vi "CRYAppend data or results file.vi"(3 "Excel path":path, 4 "Is results? (F)":bool, 5 "New/Append":string, 6 "Comment":string, 7 "Format info":T1, 8 "data format":u16, 9 "Datafile path":path, 10 "Curves list to save":string[](array[string]), 11 "Data/Wave(if true=wave)?":bool) -> (1 "error out":errorcluster)   [LabVIEW 2013]
uses:
  Data/CRYData & result stacks global.vi
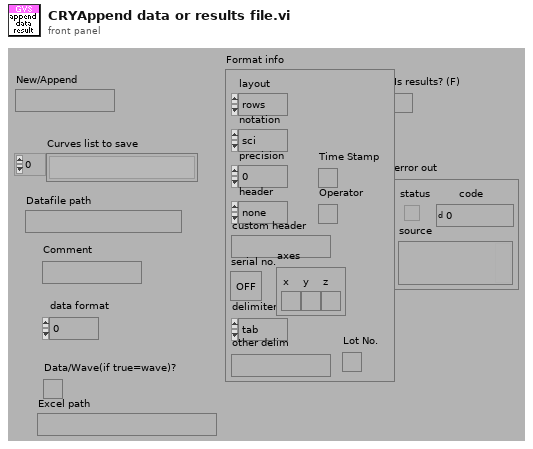
[diagram p1: front panel]
types:
  T1 = cluster{"layout":enum16{"rows", "columns"}, "notation":enum16{"sci", "float"}, "precision":i32, "header":enum16{"none", "standard", "custom"}, "custom header":string, "serial no.":bool, "delimiter":enum16{"tab", "comma", "space", "other"}, "other delim":string, "axes":cluster{"x":bool, "y":bool, "z":bool}, "Lot No.":bool, "Operator":bool, "Time Stamp":bool}
  T2 = enum16{"open", "open or create", "create or replace", "create"}
  T3 = cluster{"Datafile path":path, "file size (bytes)":i32}
  T4 = cluster{"Datafile path":path, "file size (bytes)":i32}[]
  T5 = enum16{"OK", "Yes", "YesNo", "YesNoCancel", "ReplaceAppend"}
  T6 = typedef "CRYData Cluster.ctl" = cluster{"Name":string, "Curve":cluster{"x":dbl, "y":dbl, "z":dbl}[], "X data":u16, "Y data":u16, "Z data":u16, "X axis":u16, "Y axis":u16, "Z axis":u16, "X unit":string, "Y unit":string, "Z unit":string, "X dB ref":dbl, "Y dB ref":dbl, "Z dB ref":dbl, "single val":bool, "protected":bool, "display X":bool, "display Y":bool, "display Z":bool, "Test Info":string, "Step No.":i32, "Plot Settings":cluster{"Color":u32, "Interpolation":u8, "Point Style":u8, "Line Style":u8, "Point Color":u32, "Line Width":u8, "Bar Plot Style":u8, "Fill To":i16}, "AutoProtect":bool}
  T7 = typedef "CRYResult Cluster.ctl" = cluster{"Name":string, "Margin":dbl, "unit":string, "Verdict":bool, "Limit":string, "Max/Min":string, "protected":bool, "Step No.":i32, "Test Info":string, "AutoProtect":bool}
  T8 = typedef "CRYWaveform Cluster.ctl" = cluster{"Waveform":cluster{"X0":dbl, "dX":dbl, "Y":sgl[]}, "X data":u16, "Y data":u16, "Y axis":u16, "X unit":string, "Y unit":string, "Y dB ref":dbl, "display Y":bool, "display X":bool, "Overload?":bool, "Test Info":string, "Step No.":i32, "Name":string, "protected":bool, "Sqc history":string[], "Signal Channel ID":i32, "Plot Settings":cluster{"Color":u32, "Interpolation":u8, "Point Style":u8, "Line Style":u8, "Point Color":u32, "Line Width":u8, "Bar Plot Style":u8, "Fill To":i16}, "AutoProtect":bool}
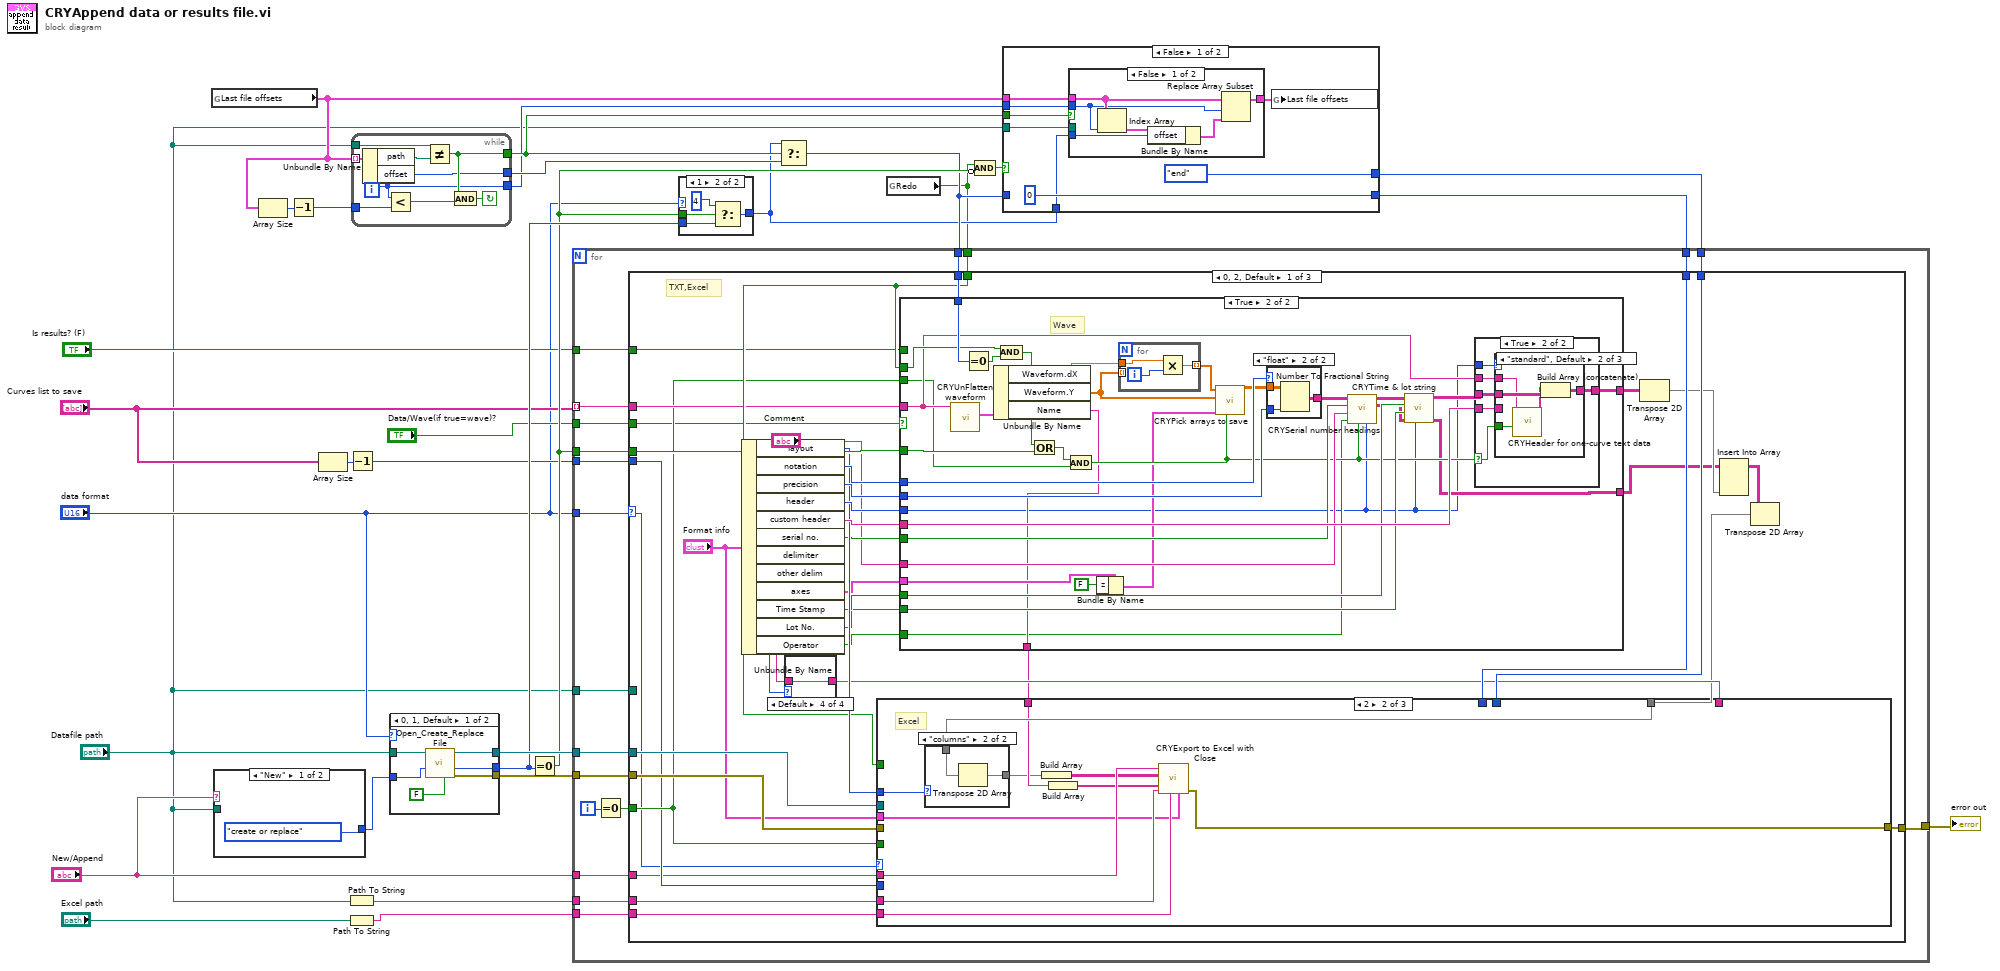
[diagram p0: block diagram]
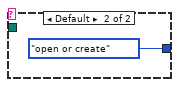
[diagram p2: hidden frame]
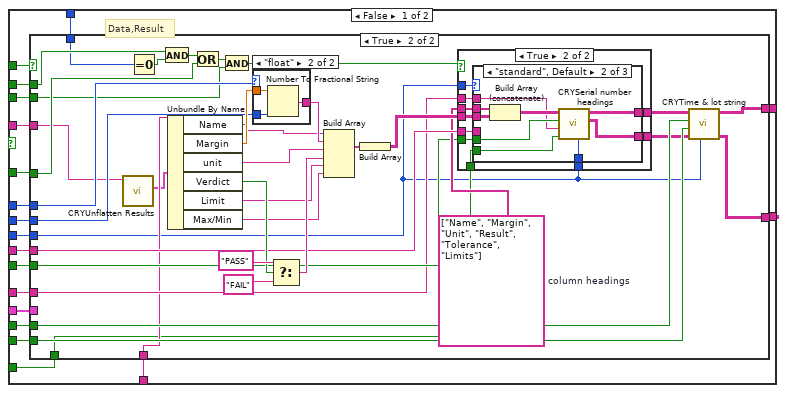
[diagram p4: hidden frame]
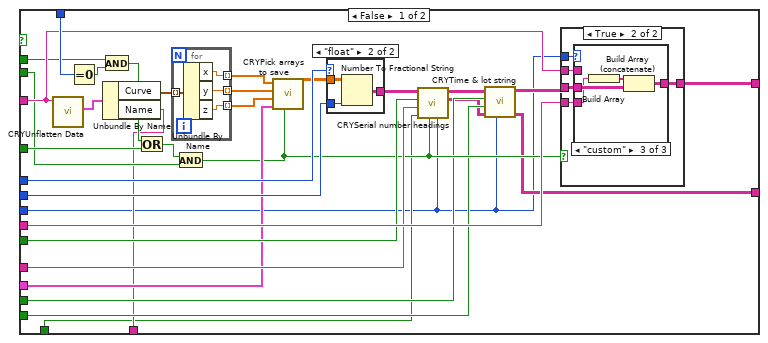
[diagram p5: hidden frame]
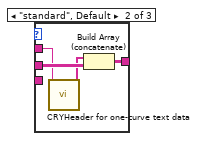
[diagram p8: hidden frame]
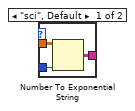
[diagram p9: hidden frame]
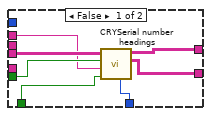
[diagram p10: hidden frame]
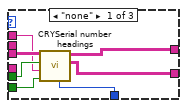
[diagram p11: hidden frame]
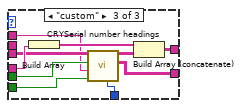
[diagram p12: hidden frame]
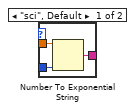
[diagram p13: hidden frame]
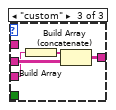
[diagram p16: hidden frame]
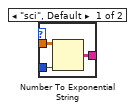
[diagram p17: hidden frame]
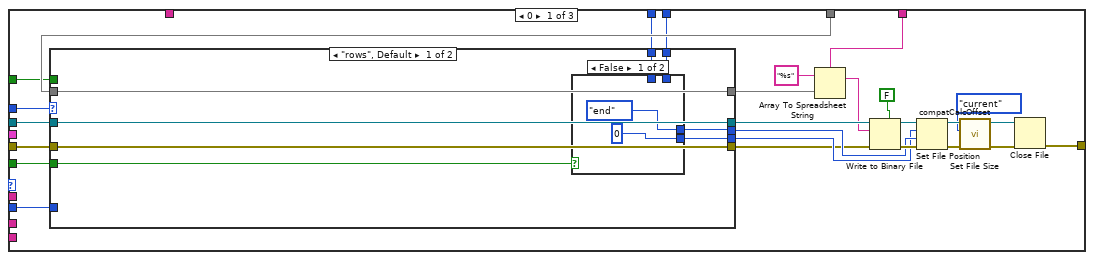
[diagram p18: hidden frame]
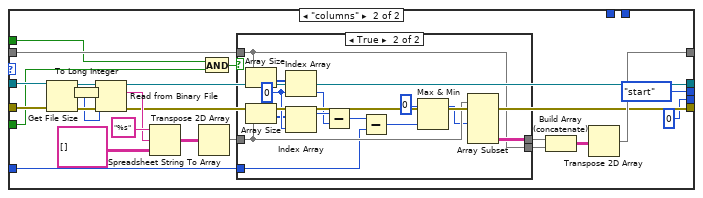
[diagram p20: hidden frame]
diagram:
  n1 = global read "CRYData & result stacks global.vi" "Last file offsets"() -> (w11:cluster{"path":path, "offset":i32}[])
  n2 = case shown="\"New\"" "New/Append" {
    tunnel: "Datafile path" -> [_ _]
    tunnel: [T2."create or replace" ("function (open:0)") T2."open or create" ("function (open:0)")] -> w1
    frame "New" {
    }
    frame Default {
    }
  }
  n3 = Array Size(array=w11) -> (size(s)=w22:i32)
  n4 = Decrement(x=w22) -> (x-1=w21:i32)
  n5 = Array Size(array="Curves list to save") -> (size(s)=w13:i32)
  n6 = Path To String(path="Datafile path") -> (string=w7:string)
  n7 = Path To String(path="Excel path") -> (string=w4:string)
  n8 = Decrement(x=w13) -> (x-1=w12:i32)
  n9 = while {
    tunnel: [w32] -> w16
    tunnel: "Datafile path" -> [w33]
    tunnel: [w34] -> w19
    tunnel: [w37] -> w17
    tunnel: w21 -> [w40]
    tunnel: w11 -> [w39] mode=indexing
    i -> [w32]
    stop <- w35 continue-if-true
    n10 = Unbundle By Name(w39) -> ("path"=w38:path, "offset"=w34:i32)
    n11 = Less?(x=w32, y=w40) -> (x < y?=w36:bool)
    n12 = Not Equal?(x=w33, y=w38) -> (x != y?=w37:bool)
    n13 = And(x=w37, y=w36) -> (x .and. y?=w35:bool)
  }
  n14 = case shown="0, 1, Default" "data format" {
    tunnel: w1 -> [w46 _]
    tunnel: [w45 _] -> w28
    tunnel: [w44 _] -> w27
    tunnel: [w43 _] -> w26
    tunnel: "Datafile path" -> [w42 _]
    frame 0, 1, Default {
      n15 = call <vilib>:"Open_Create_Replace File.vi"("advisory dialog? (display:T)"=FALSE, "function (open:0)"=w46, "file path"=w42) -> ("error out"=w44:errorcluster, "file size (bytes)"=w43:i32, "refnum"=w45:refnum<file>)  [unwired: 4 in, 2 out]
    }
    frame 2, 3 {
    }
  }
  n16 = Equal To 0?(x=w26) -> (x = 0?=w25:bool)
  n17 = case shown="1" "data format" {
    tunnel: w26 -> [w47 w50]
    tunnel: w25 -> [_ w49]
    tunnel: [w47 w48] -> w15
    frame 0, 2, Default {
    }
    frame 1 {
      n18 = Select(t=4, s=w49, f=w50) -> (s? t:f=w48:i32)
    }
  }
  n19 = Select(t=w15, s=w17, f=w19) -> (s? t:f=w18:i32)
  n20 = global read "CRYData & result stacks global.vi" "Redo"() -> (w10:bool)
  n21 = Compound Arithmetic op=AND(w10, invert w25) -> (w29:bool)
  n22 = case shown="False" w29 {
    tunnel: [enum16{"start", "end", "current"}."end" ("pos mode (0:2)") enum16{"start", "end", "current"}."start" ("pos mode (0:2)")] -> w24
    tunnel: [0 ("pos offset (0)") w71] -> w23
    tunnel: w18 -> [_ w71]
    tunnel: w15 -> [w54 _]
    tunnel: w17 -> [w57 _]
    tunnel: w11 -> [w56 _]
    tunnel: w16 -> [w55 _]
    tunnel: "Datafile path" -> [w53 _]
    frame False {
      n23 = case shown="False" w57 {
        tunnel: w56 -> [w63 w68]
        tunnel: w55 -> [w60 _]
        tunnel: w54 -> [w65 w70]
        tunnel: [w61 w67] -> w52
        tunnel: w53 -> [_ w66]
        frame False {
          n24 = Index Array(array=w63, index=w60) -> (element=w64:cluster{"path":path, "offset":i32})
          n25 = Bundle By Name(cluster=w64, "offset"=w65) -> (w62:cluster{"path":path, "offset":i32})
          n26 = Replace Array Subset(array=w63, new element=w62, index=w60) -> (w61:cluster{"path":path, "offset":i32}[])
        }
        frame True {
          n27 = Bundle("Datafile path"=w66, "file size (bytes)"=w70) -> (w69:T3)  [unwired: 1 out]
          n28 = Build Array (concatenate)(w68, w69) -> (w67:T4)
        }
      }
      n29 = global write "CRYData & result stacks global.vi" "Last file offsets"(w52) -> ()
    }
    frame True {
    }
  }
  n30 = for {
    tunnel: w10 -> [w91]
    tunnel: "Curves list to save" -> [w90] mode=indexing
    tunnel: w28 -> [w89]
    tunnel: w27 -> [w88]
    tunnel: w25 -> [w87]
    tunnel: w24 -> [w86]
    tunnel: w23 -> [w85]
    tunnel: "data format" -> [w84]
    tunnel: "Is results? (F)" -> [w83]
    tunnel: w18 -> [w82]
    tunnel: [w78] -> w9
    tunnel: w12 -> [w79]
    tunnel: "Datafile path" -> [w77]
    tunnel: "Data/Wave(if true=wave)?" -> [w76]
    tunnel: w7 -> [w75]
    tunnel: "New/Append" -> [w74]
    tunnel: w4 -> [w73]
    i -> [w81]
    n31 = Equal To 0?(x=w81) -> (x = 0?=w80:bool)
    n32 = case shown="0, 2, Default" w84 {
      selector: w84 -> [w103 _ _]
      tunnel: w90 -> [w111 w471 w517]
      tunnel: w82 -> [w129 w477 _]
      tunnel: w91 -> [w118 w472 _]
      tunnel: w87 -> [w128 w476 _]
      tunnel: w89 -> [w123 w474 _]
      tunnel: [w105 w449 errorcluster {"status"=FALSE, "code"=0, "source"=""} ("error out")] -> w78
      tunnel: w88 -> [w122 w473 _]
      tunnel: w86 -> [w120 w468 _]
      tunnel: w85 -> [w119 w467 _]
      tunnel: w83 -> [w117 _ _]
      tunnel: w80 -> [w110 w466 _]
      tunnel: w79 -> [w109 _ _]
      tunnel: w77 -> [_ _ w515]
      tunnel: w76 -> [w104 _ _]
      tunnel: w75 -> [w102 _ _]
      tunnel: w74 -> [w100 _ _]
      tunnel: w73 -> [w99 _ _]
      frame 0, 2, Default {
        # "TXT,Excel"
        n33 = Unbundle By Name("Format info") -> ("layout"=w121:enum16{"rows", "columns"}, "notation"=w126:enum16{"sci", "float"}, "precision"=w127:i32, "header"=w125:enum16{"none", "standard", "custom"}, "custom header"=w124:string, "serial no."=w116:bool, "delimiter"=w114:enum16{"tab", "comma", "space", "other"}, "other delim"=w113:string, "axes"=w108:cluster{"x":bool, "y":bool, "z":bool}, "Time Stamp"=w107:bool, "Lot No."=w106:bool, "Operator"=w93:bool)
        n34 = case shown="Default" w114 {
          tunnel: w113 -> [_ _ _ w448]
          tunnel: ["\t" "," " " w448] -> w112
          frame "tab" {
          }
          frame "comma" {
          }
          frame "space" {
          }
          frame Default {
          }
        }
        n35 = case shown="True" w104 {
          tunnel: w129 -> [w148 w323]
          tunnel: w128 -> [w147 w322]
          tunnel: w127 -> [w146 w321]
          tunnel: w126 -> [w145 w320]
          tunnel: w125 -> [w144 w291]
          tunnel: w124 -> [w143 w319]
          tunnel: [w142 w318] -> w97
          tunnel: w118 -> [w141 w317]
          tunnel: w117 -> [w140 _]
          tunnel: w116 -> [w139 w316]
          tunnel: "Comment" -> [w138 w315]
          tunnel: w111 -> [w137 w314]
          tunnel: w110 -> [w136 w313]
          tunnel: w108 -> [w135 w301]
          tunnel: w107 -> [w134 w312]
          tunnel: w106 -> [w133 w311]
          tunnel: [w132 w295] -> w101
          tunnel: [w131 w293] -> w94
          tunnel: w93 -> [w130 w292]
          frame False {
            # "Data,Result"
            n36 = case shown="True" w140 {
              tunnel: w148 -> [w178 w227]
              tunnel: w147 -> [w175 w226]
              tunnel: w146 -> [w174 w224]
              tunnel: w145 -> [w173 w223]
              tunnel: w144 -> [w149 w206]
              tunnel: w143 -> [w172 w231]
              tunnel: w138 -> [w167 w213]
              tunnel: w137 -> [w171 w211]
              tunnel: [w152 w214] -> w142
              tunnel: w141 -> [w170 w228]
              tunnel: w139 -> [w168 w222]
              tunnel: w136 -> [w166 w221]
              tunnel: w135 -> [w161 _]
              tunnel: w134 -> [w158 w216]
              tunnel: w133 -> [w157 w215]
              tunnel: [w155 w212] -> w132
              tunnel: [w151 w208] -> w131
              tunnel: w130 -> [w150 w207]
              frame False {
                n37 = call "CRYUnflatten Data.vi"("Unflatten data"=w171) -> ("Datum"=w176:T6)  [unwired: 8 in, 2 out]
                n38 = Equal To 0?(x=w178) -> (x = 0?=w179:bool)
                n39 = And(x=w170, y=w179) -> (x .and. y?=w180:bool)
                n40 = Unbundle By Name(w176) -> ("Curve"=w177:cluster{"x":dbl, "y":dbl, "z":dbl}[], "Name"=w155:string)
                n41 = Or(x=w180, y=w175) -> (x .or. y?=w165:bool)
                n42 = for {
                  tunnel: w177 -> [w205] mode=indexing
                  tunnel: [w204] -> w164 mode=indexing
                  tunnel: [w203] -> w163 mode=indexing
                  tunnel: [w202] -> w162 mode=indexing
                  n43 = Unbundle By Name(w205) -> ("x"=w204:dbl, "y"=w203:dbl, "z"=w202:dbl)
                }
                n44 = And(x=w165, y=w166) -> (x .and. y?=w159:bool)
                n45 = call "CRYPick arrays to save.vi"("Start of file"=w159, "axes"=w161, "Z"=w162, "Y"=w163, "X"=w164) -> ("Data points to save"=w160:dbl[][])  [unwired: 6 in]
                n46 = case shown="\"float\"" w173 {
                  tunnel: w160 -> [w198 w201]
                  tunnel: w174 -> [w197 w200]
                  tunnel: [w196 w199] -> w169
                  frame "sci", Default {
                    n47 = Number To Exponential String(number=w198, precision (6)=w197) -> (E-format string=w196:string[][])  [unwired: 2 out]
                  }
                  frame "float" {
                    n48 = Number To Fractional String(number=w201, precision (6)=w200) -> (F-format string=w199:string[][])  [unwired: 2 out]
                  }
                }
                n49 = call "CRYSerial number headings.vi"("header"=w149, "Start of file"=w159, "Operator"=w150, "Comment"=w167, "Include serial numbers (F)"=w168, "Table in"=w169) -> ("Header out"=w153:string[][], "Table out"=w154:string[][])  [unwired: 4 in]
                n50 = call "CRYTime & lot string.vi"("header"=w149, "Header in"=w153, "Lot No."=w157, "Time Stamp"=w158, "Table in"=w154) -> ("Header out"=w151:string[][], "Table out"=w156:string[][])  [unwired: 3 in, 2 out]
                n51 = case shown="True" w159 {
                  tunnel: w149 -> [_ w186]
                  tunnel: w172 -> [_ w185]
                  tunnel: w171 -> [_ w184]
                  tunnel: [w181 w183] -> w152
                  tunnel: w156 -> [w181 w182]
                  frame False {
                  }
                  frame True {
                    n52 = case shown="\"custom\"" w186 {
                      tunnel: w182 -> [w187 w191 w195]
                      tunnel: [w187 w190 w194] -> w183
                      tunnel: w185 -> [_ _ w193]
                      tunnel: w184 -> [_ w188 _]
                      frame "none" {
                      }
                      frame "standard", Default {
                        n53 = call "CRYHeader for one-curve text data.vi"("Data curve, flat"=w188) -> ("Header row"=w189:string[])  [unwired: 10 in]
                        n54 = Build Array (concatenate)(w189, w191) -> (w190:string[][])
                      }
                      frame "custom" {
                        n55 = Build Array(w193) -> (w192:string[])
                        n56 = Build Array (concatenate)(w192, w195) -> (w194:string[][])
                      }
                    }
                  }
                }
              }
              frame True {
                w230 = string[] ["Name", "Margin", "Unit", "Result", "Tolerance", "Limits"]  # column headings
                n57 = call "CRYUnflatten Results.vi"("Unflatten Result"=w211) -> ("Result"=w210:T7)  [unwired: 8 in, 2 out]
                n58 = Equal To 0?(x=w227) -> (x = 0?=w229:bool)
                n59 = And(x=w228, y=w229) -> (x .and. y?=w225:bool)
                n60 = Unbundle By Name(w210) -> ("Name"=w212:string, "Margin"=w236:dbl, "unit"=w218:string, "Verdict"=w239:bool, "Limit"=w237:string, "Max/Min"=w234:string)
                n61 = Or(x=w225, y=w226) -> (x .or. y?=w220:bool)
                n62 = And(x=w220, y=w221) -> (x .and. y?=w219:bool)
                n63 = case shown="\"float\"" w223 {
                  tunnel: w236 -> [w287 w290]
                  tunnel: w224 -> [w286 w289]
                  tunnel: [w285 w288] -> w235
                  frame "sci", Default {
                    n64 = Number To Exponential String(number=w287, precision (6)=w286) -> (E-format string=w285:string)  [unwired: 2 out]
                  }
                  frame "float" {
                    n65 = Number To Fractional String(number=w290, precision (6)=w289) -> (F-format string=w288:string)  [unwired: 2 out]
                  }
                }
                n66 = Select(t="PASS", s=w239, f="FAIL") -> (s? t:f=w238:string)
                n67 = Build Array(w212, w235, w218, w238, w237, w234) -> (w233:string[])
                n68 = Build Array(w233) -> (w232:string[][])
                n69 = case shown="True" w219 {
                  tunnel: w232 -> [w248 w258]
                  tunnel: [w247 w257] -> w217
                  tunnel: w230 -> [_ w256]
                  tunnel: w213 -> [w245 w255]
                  tunnel: w231 -> [_ w254]
                  tunnel: w206 -> [_ w253]
                  tunnel: w222 -> [w246 w252]
                  tunnel: [w244 w251] -> w209
                  tunnel: w207 -> [w243 w250]
                  tunnel: w206 -> [w242 w249]
                  frame False {
                    n70 = call "CRYSerial number headings.vi"("header"=w242, "Operator"=w243, "Comment"=w245, "Include serial numbers (F)"=w246, "Table in"=w248) -> ("Header out"=w244:string[][], "Table out"=w247:string[][])  [unwired: 5 in]
                  }
                  frame True {
                    n71 = case shown="\"standard\", Default" w253 {
                      tunnel: w256 -> [_ w274 _]
                      tunnel: w258 -> [w265 w273 w281]
                      tunnel: [w264 w271 w284] -> w257
                      tunnel: w254 -> [_ _ w283]
                      tunnel: w255 -> [w262 w269 w278]
                      tunnel: w252 -> [w263 w270 w279]
                      tunnel: [w261 w268 w277] -> w251
                      tunnel: w250 -> [w260 w267 w276]
                      tunnel: w249 -> [w259 w266 w275]
                      frame "none" {
                        n72 = call "CRYSerial number headings.vi"("header"=w259, "Operator"=w260, "Comment"=w262, "Include serial numbers (F)"=w263, "Table in"=w265) -> ("Header out"=w261:string[][], "Table out"=w264:string[][])  [unwired: 5 in]
                      }
                      frame "standard", Default {
                        n73 = Build Array (concatenate)(w274, w273) -> (w272:string[][])
                        n74 = call "CRYSerial number headings.vi"("header"=w266, "Operator"=w267, "Comment"=w269, "Include serial numbers (F)"=w270, "Table in"=w272) -> ("Header out"=w268:string[][], "Table out"=w271:string[][])  [unwired: 5 in]
                      }
                      frame "custom" {
                        n75 = Build Array(w283) -> (w282:string[])
                        n76 = call "CRYSerial number headings.vi"("header"=w275, "Operator"=w276, "Comment"=w278, "Include serial numbers (F)"=w279, "Table in"=w281) -> ("Header out"=w277:string[][], "Table out"=w280:string[][])  [unwired: 5 in]
                        n77 = Build Array (concatenate)(w282, w280) -> (w284:string[][])
                      }
                    }
                  }
                }
                n78 = call "CRYTime & lot string.vi"("header"=w206, "Header in"=w209, "Lot No."=w215, "Time Stamp"=w216, "Table in"=w217) -> ("Header out"=w208:string[][], "Table out"=w214:string[][])  [unwired: 3 in, 2 out]
              }
            }
          }
          frame True {
            # "Wave"
            n79 = call "CRYUnFlatten waveform.vi"("Unflatten Waveform"=w314) -> ("Waveform Cluster"=w308:T8)  [unwired: 8 in, 2 out]
            n80 = Equal To 0?(x=w323) -> (x = 0?=w309:bool)
            n81 = Unbundle By Name(w308) -> ("Waveform.dX"=w297:dbl, "Waveform.Y"=w298:sgl[], "Name"=w295:string)
            n82 = And(x=w317, y=w309) -> (x .and. y?=w310:bool)
            n83 = Or(x=w310, y=w322) -> (x .or. y?=w306:bool)
            n84 = And(x=w306, y=w313) -> (x .and. y?=w304:bool)
            n85 = Bundle By Name(cluster=w301, "z"=FALSE) -> (w299:cluster{"x":bool, "y":bool, "z":bool})
            n86 = for {
              tunnel: w298 -> [_] mode=indexing
              tunnel: w297 -> [w325]
              tunnel: [w324] -> w296 mode=indexing
              i -> [w326]
              n87 = Multiply(x=w325, y=w326) -> (x*y=w324:dbl)
            }
            n88 = call "CRYPick arrays to save.vi"("Start of file"=w304, "axes"=w299, "Y"=w298, "X"=w296) -> ("Data points to save"=w305:dbl[][])  [unwired: 7 in]
            n89 = case shown="\"float\"" w320 {
              tunnel: w305 -> [w346 w349]
              tunnel: w321 -> [w345 w348]
              tunnel: [w344 w347] -> w307
              frame "sci", Default {
                n90 = Number To Exponential String(number=w346, precision (6)=w345) -> (E-format string=w344:string[][])  [unwired: 2 out]
              }
              frame "float" {
                n91 = Number To Fractional String(number=w349, precision (6)=w348) -> (F-format string=w347:string[][])  [unwired: 2 out]
              }
            }
            n92 = call "CRYSerial number headings.vi"("header"=w291, "Start of file"=w304, "Operator"=w292, "Comment"=w315, "Include serial numbers (F)"=w316, "Table in"=w307) -> ("Header out"=w294:string[][], "Table out"=w303:string[][])  [unwired: 4 in]
            n93 = call "CRYTime & lot string.vi"("header"=w291, "Header in"=w294, "Lot No."=w311, "Time Stamp"=w312, "Table in"=w303) -> ("Header out"=w293:string[][], "Table out"=w302:string[][])  [unwired: 3 in, 2 out]
            n94 = case shown="True" w304 {
              selector: w304 -> [_ w328]
              tunnel: w291 -> [_ w333]
              tunnel: w319 -> [_ w332]
              tunnel: w314 -> [_ w331]
              tunnel: [w327 w330] -> w318
              tunnel: w302 -> [w327 w329]
              frame False {
              }
              frame True {
                n95 = case shown="\"standard\", Default" w333 {
                  tunnel: w329 -> [w334 w339 w343]
                  tunnel: [w334 w338 w342] -> w330
                  tunnel: w332 -> [_ _ w341]
                  tunnel: w331 -> [_ w336 _]
                  tunnel: w328 -> [_ w335 _]
                  frame "none" {
                  }
                  frame "standard", Default {
                    n96 = call "CRYHeader for one-curve text data.vi"("Data/Wave(if true=wave)?"=w335, "Data curve, flat"=w336) -> ("Header row"=w337:string[])  [unwired: 9 in]
                    n97 = Build Array (concatenate)(w337, w339) -> (w338:string[][])
                  }
                  frame "custom" {
                    n98 = Build Array(w341) -> (w340:string[])
                    n99 = Build Array (concatenate)(w340, w343) -> (w342:string[][])
                  }
                }
              }
            }
          }
        }
        n100 = Transpose 2D Array(2D array=w97) -> (transposed array=w96:string[][])
        n101 = Insert Into Array(array=w94, new element=w96) -> (w98:string[][])  [unwired: 2 in]
        n102 = Transpose 2D Array(2D array=w98) -> (transposed array=w95:string[][])
        n103 = case shown="2" w103 {
          tunnel: w123 -> [w378 _ _]
          tunnel: w122 -> [w377 _ _]
          tunnel: w121 -> [w376 w430 _]
          tunnel: w95 -> [w375 w440 _]
          tunnel: w120 -> [w373 _ _]
          tunnel: w119 -> [w372 _ _]
          tunnel: w118 -> [w371 _ _]
          tunnel: w112 -> [w370 _ _]
          tunnel: w110 -> [w369 _ _]
          tunnel: w109 -> [w368 _ _]
          tunnel: [w350 w437 errorcluster {"status"=FALSE, "code"=0, "source"=""} ("error out")] -> w105
          tunnel: w102 -> [_ w438 _]
          tunnel: w101 -> [_ w439 _]
          tunnel: w100 -> [_ w436 _]
          tunnel: w99 -> [_ w433 _]
          tunnel: "Format info" -> [_ w431 _]
          frame 0 {
            n104 = case shown="\"rows\", Default" w376 {
              tunnel: [w386 w402] -> w357
              tunnel: w378 -> [w386 w414]
              tunnel: [w385 w403] -> w354
              tunnel: w377 -> [w385 w413]
              tunnel: w375 -> [w384 w399]
              tunnel: [w384 w404] -> w367
              tunnel: w373 -> [w383 _]
              tunnel: [w381 enum16{"start", "end", "current"}."start" ("pos mode (0:2)")] -> w356
              tunnel: w372 -> [w382 _]
              tunnel: [w380 0] -> w355
              tunnel: w371 -> [_ w394]
              tunnel: w369 -> [w379 w393]
              tunnel: w368 -> [_ w395]
              frame "rows", Default {
                n105 = case shown="False" w379 {
                  tunnel: w383 -> [_ w390]
                  tunnel: w382 -> [_ w389]
                  tunnel: [enum16{"start", "end", "current"}."end" ("pos mode (0:2)") w390] -> w381
                  tunnel: [0 ("pos offset (0)") w389] -> w380
                  frame False {
                  }
                  frame True {
                  }
                }
              }
              frame "columns" {
                n106 = Get File Size(file=w414, error in=w413) -> (refnum out=w412:refnum<file>, size (in bytes)=w391:i64, 0:w411:errorcluster)
                n107 = To Long Integer(number=w391) -> (32bit integer=w410:i32)
                n108 = Read from Binary File(8:w411, 10:w410, 11:w412) -> (0:w403:errorcluster, 2:w408:string, 3:w402:refnum<file>)  [unwired: 4 out]
                n109 = Spreadsheet String To Array(format string="%s", spreadsheet string=w408, array type (2D Dbl)=string[][] []) -> (array=w406:string[][])  [unwired: 1 out]
                n110 = Transpose 2D Array(2D array=w406) -> (transposed array=w396:string[][])
                n111 = And(x=w394, y=w393) -> (x .and. y?=w392:bool)
                n112 = case shown="True" w392 {
                  tunnel: [w416 w422] -> w398
                  tunnel: w399 -> [w416 w422]
                  tunnel: w396 -> [w415 w424]
                  tunnel: [w415 w423] -> w397
                  tunnel: w395 -> [_ w417]
                  frame False {
                  }
                  frame True {
                    w429 = 0
                    n113 = Array Size(array=w422) -> (size(s)=w427:i32[])
                    n114 = Array Size(array=w424) -> (size(s)=w428:i32[])
                    n115 = Index Array(array=w427, index=w429) -> (element=w425:i32)
                    n116 = Index Array(array=w428, index=w429) -> (element=w426:i32)
                    n117 = Subtract(x=w426, y=w425) -> (x-y=w419:i32)
                    n118 = Subtract(x=w419, y=w417) -> (x-y=w418:i32)
                    n119 = Max & Min(x=0, y=w418) -> (max(x,y)=w421:i32)  [unwired: 1 out]
                    n120 = Array Subset(array=w424, length (row)=w421) -> (w423:string[][])  [unwired: 3 in]
                  }
                }
                n121 = Build Array (concatenate)(w397, w398) -> (w405:string[][])
                n122 = Transpose 2D Array(2D array=w405) -> (transposed array=w404:string[][])
              }
            }
            n123 = Array To Spreadsheet String(delimiter (Tab)=w370, array=w367, 3:"%s") -> (spreadsheet string=w353:string)
            n124 = Set File Position(offset (in bytes) (0)=w355, refnum=w357, from (0:start)=w356, error in=w354) -> (refnum out=w364:refnum<file>, error out=w365:errorcluster)
            n125 = Write to Binary File(file (use dialog)=w364, data=w353, error in=w365, 5:FALSE ("预置数组或字符串大小？(T)")) -> (refnum out=w359:refnum<file>, error out=w360:errorcluster)  [unwired: 3 out]
            n126 = call <vilib>:"compatCalcOffset.vi"("error in"=w360, "pos mode (0:1)"=enum16{"start", "end", "current"}."current", "refnum"=w359) -> ("error out"=w361:errorcluster, "offset"=w362:i32, "dup refnum"=w363:refnum<file>)  [unwired: 1 in, 5 out]
            n127 = Set File Size(4:w361, 6:w362, 7:w363) -> (0:w351:errorcluster, 3:w352:refnum<file>)
            n128 = Close File(refnum=w352, error in=w351) -> (error out=w350:errorcluster)  [unwired: 1 out]
          }
          frame 2 {
            # "Excel"
            n129 = case shown="\"columns\"" w430 {
              tunnel: w440 -> [w441 w443]
              tunnel: [w441 w442] -> w432
              frame "rows", Default {
              }
              frame "columns" {
                n130 = Transpose 2D Array(2D array=w443) -> (transposed array=w442:string[][])
              }
            }
            n131 = Build Array(w432) -> (w434:string[][][])
            n132 = Build Array(w439) -> (w435:string[])
            n133 = call "CRYExport to Excel with Close.vi"("Format info"=w431, "ExcelPath"=w433, "FilePath"=w438, "Sheet Names"=w435, "Data"=w434, "New/Append"=w436) -> ("error out"=w437:errorcluster)  [unwired: 5 in]
          }
          frame 1, Default {
          }
        }
      }
      frame 1 {
        # "DAT,WFM"
        n134 = Equal To 0?(x=w477) -> (x = 0?=w478:bool)
        n135 = And(x=w472, y=w478) -> (x .and. y?=w475:bool)
        n136 = Or(x=w475, y=w476) -> (x .or. y?=w470:bool)
        n137 = And(x=w470, y=w466) -> (x .and. y?=w469:bool)
        n138 = case shown="False" w469 {
          tunnel: w474 -> [w487 w509]
          tunnel: w473 -> [w486 w510]
          tunnel: [w484 w511] -> w453
          tunnel: [w485 w512] -> w452
          tunnel: w472 -> [w483 _]
          frame False {
            n139 = case shown="True" w483 {
              tunnel: w487 -> [w502 w504]
              tunnel: w486 -> [w501 w503]
              tunnel: [w491 w504] -> w485
              tunnel: [w492 w503] -> w484
              frame False {
                w497 = 0
                w500 = 1  # count
                n140 = Read from Binary File(5:w497, 8:w501, 10:w500, 11:w502) -> (0:w494:errorcluster, 2:w499:i32[], 3:w495:refnum<file>)  [unwired: 3 out]
                n141 = Index Array(array=w499, index=w497) -> (element=w498:i32)
                n142 = Increment(x=w498) -> (x+1=w493:i32)
                n143 = Set File Position(refnum=w495, from (0:start)=enum16{"start", "end", "current"}."start" ("pos mode (0:2)"), error in=w494) -> (refnum out=w490:refnum<file>, error out=w489:errorcluster)  [unwired: 1 out]
                n144 = Write to Binary File(file (use dialog)=w490, data=w493, error in=w489, 5:FALSE ("预置数组或字符串大小？(T)")) -> (refnum out=w491:refnum<file>, error out=w492:errorcluster)  [unwired: 3 out]
              }
              frame True {
              }
            }
          }
          frame True {
            n145 = Set File Position(refnum=w509, from (0:start)=enum16{"start", "end", "current"}."start" ("pos mode (0:2)"), error in=w510) -> (refnum out=w507:refnum<file>, error out=w506:errorcluster)  [unwired: 1 out]
            n146 = Write to Binary File(file (use dialog)=w507, data=1, error in=w506, 5:FALSE ("预置数组或字符串大小？(T)")) -> (refnum out=w512:refnum<file>, error out=w511:errorcluster)  [unwired: 3 out]
          }
        }
        n147 = Flatten To String(anything=w471) -> (data string=w456:string)  [unwired: 1 in, 4 out]
        n148 = case shown="True" w466 {
          tunnel: w468 -> [_ w482]
          tunnel: [enum16{"start", "end", "current"}."end" ("pos mode (0:2)") w482] -> w455
          tunnel: [0 ("pos offset (0)") w481] -> w454
          tunnel: w467 -> [_ w481]
          frame False {
          }
          frame True {
          }
        }
        n149 = Set File Position(offset (in bytes) (0)=w454, refnum=w452, from (0:start)=w455, error in=w453) -> (refnum out=w463:refnum<file>, error out=w464:errorcluster)
        n150 = Write to Binary File(file (use dialog)=w463, data=w456, error in=w464, 5:FALSE ("预置数组或字符串大小？(T)")) -> (refnum out=w458:refnum<file>, error out=w459:errorcluster)  [unwired: 3 out]
        n151 = call <vilib>:"compatCalcOffset.vi"("error in"=w459, "pos mode (0:1)"=enum16{"start", "end", "current"}."current", "refnum"=w458) -> ("error out"=w460:errorcluster, "offset"=w461:i32, "dup refnum"=w462:refnum<file>)  [unwired: 1 in, 5 out]
        n152 = Set File Size(4:w460, 6:w461, 7:w462) -> (0:w450:errorcluster, 3:w451:refnum<file>)
        n153 = Close File(refnum=w451, error in=w450) -> (error out=w449:errorcluster)  [unwired: 1 out]
      }
      frame 3 {
        # "Wave"
        n154 = call "CRYUnFlatten waveform.vi"("Unflatten Waveform"=w517) -> ("Waveform Cluster"=w516:T8)  [unwired: 8 in, 2 out]
        n155 = Unbundle By Name(w516) -> ("Waveform.dX"=w522:dbl, "Waveform.Y"=w520:sgl[])
        n156 = Reciprocal(x=w522) -> (1/x=w521:dbl)
        n157 = call "CRYSave Wave File.vi"("Channel"=u32 1, "Wave Data In"=w520, "Sampling Freq"=w521, "Wave File Path In"=w515) -> ("Error Out(0-OK)"=w519:u32)  [unwired: 7 in]
        n158 = case shown="Default" w519 {
          frame Default {
            n159 = call "CRYGet Error Message.vi"("Error No"=4, "Kind"="Curves Library") -> ("Message"=w524:string, "Window Title"=w525:string)  [unwired: 4 in, 4 out]
            n160 = call "CRYMessage Dialog.vi"("Window Title"=w525, "YesNoCancel"=T5."OK", "Message Content"=w524) -> ()  [unwired: 7 in, 2 out]
          }
          frame 0 {
          }
        }
      }
    }
  }
  "error out" <- w9
